vi "Update Kitchen Fire And Duration.vi"(8 "error in (no error)":errorcluster, 9 "Timer (s)":dbl, 10 "Fire (%)":dbl, 11 "COOKING in":refnum<class "COOKING.lvclass">) -> (0 "error out":errorcluster, 3 "COOKING out":refnum<class "COOKING.lvclass">)   [LabVIEW 2024, in "Chef States.lvlib" / "COOKING.lvclass"]
uses:
  COOKING.lvclass
  COOKING.lvclass/COOKING.ctl
  Kitchen Actor Messages/Update Fire Msg/Update Fire Msg.lvclass
  Kitchen Actor Messages/Update Timer Msg/Update Timer Msg.lvclass
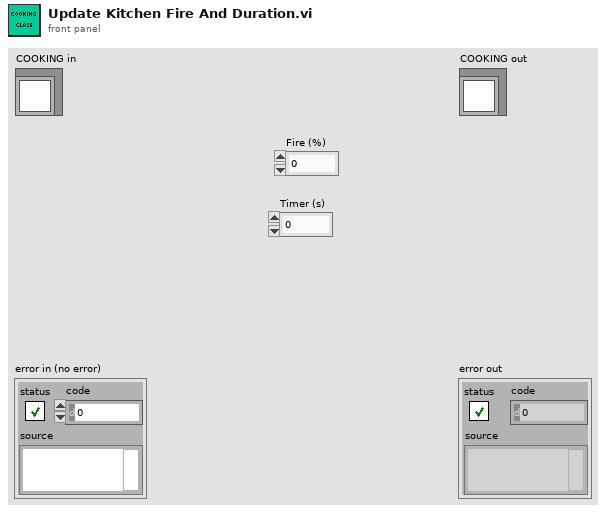
[diagram p1: front panel]
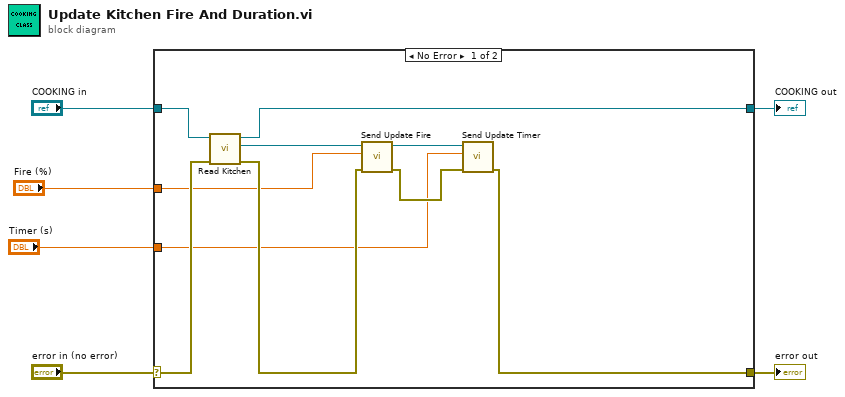
[diagram p0: block diagram]
diagram:
  n1 = case shown="No Error" "error in (no error)" {
    selector: "error in (no error)" -> [w15 w18]
    tunnel: [w9 w18] -> w5
    tunnel: [w14 w17] -> w3
    tunnel: "COOKING in" -> [w16 w17]
    tunnel: "Fire (%)" -> [w8 _]
    tunnel: "Timer (s)" -> [w7 _]
    frame No Error {
      n2 = call-dynamic "Read Kitchen.vi"("error in (no error)"=w15, "COOKING in"=w16) -> ("error out"=w10:errorcluster, "Kitchen"=w13:refnum<class "Message Enqueuer.lvclass">, "COOKING out"=w14:refnum<class "COOKING.lvclass">)  [unwired: 7 in]
      n3 = call "Send Update Fire.vi"("error in (no error)"=w10, "Fire (%)"=w8, "Message Enqueuer"=w13) -> ("error out"=w11:errorcluster, "Message Enqueuer out"=w12:refnum<class "Message Enqueuer.lvclass">)  [unwired: 7 in]
      n4 = call "Send Update Timer.vi"("error in (no error)"=w11, "Timer (s)"=w7, "Message Enqueuer"=w12) -> ("error out"=w9:errorcluster)  [unwired: 7 in, 1 out]
    }
    frame Error {
    }
  }
  "error out" <- w5
  "COOKING out" <- w3
